vi "CallingRustDLL.vi"() -> ()   [LabVIEW 2018]
uses:
  Desktop/LabViewWorks/rust_labview_basic.dll
panel:
  out "return":i32
  in  "value":i32
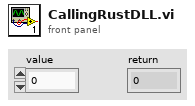
[diagram p1: front panel]
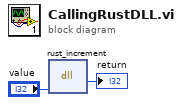
[diagram p0: block diagram]
diagram:
  n1 = dll-call lib="C:/Users/user/Desktop/LabViewWorks/rust_labview_basic.dll" fn="rust_increment"("value"="value") -> ("return"=→"return":i32)  [unwired: 4 in, 2 out]
